vi "writeAPDInfo.vi"(8 "error in (no error)":errorcluster, 9 "iRF Data":cluster{"dt":dbl, "Ctrl V":dbl[], "iRF":dbl[][]}={"dt"=0.0, "Ctrl V"=[0.0], "iRF"=[[0.0]]}, 10 "Gain Data":cluster{"CtrlV":dbl[], "Gain":dbl[]}={"CtrlV"=[0.0], "Gain"=[0.0]}, 11 "APD Serial #":string) -> (0 "error out (no error)":errorcluster)   [LabVIEW 2020]
panel:
  out "appended path":path
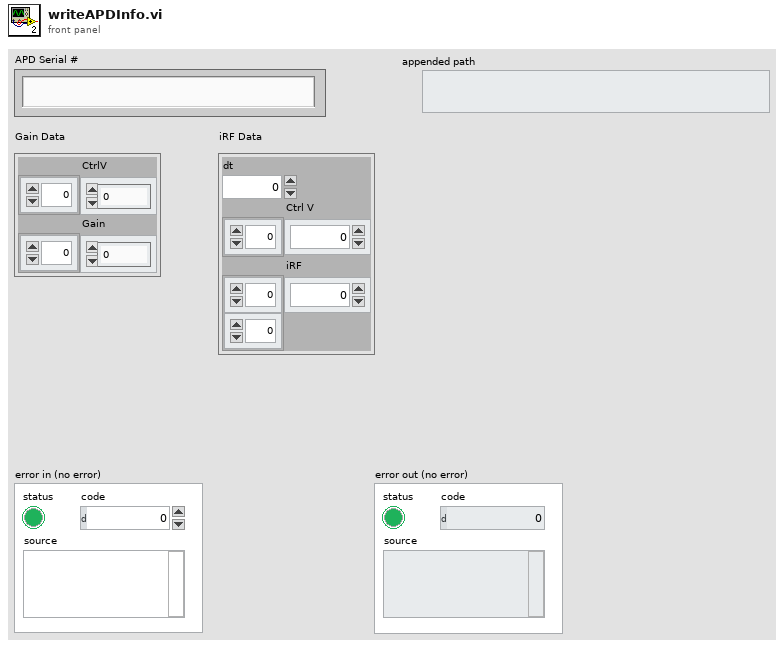
[diagram p1: front panel]
types:
  T1 = enum16{"open", "open or create", "create or replace", "create", "open (read-only)"}
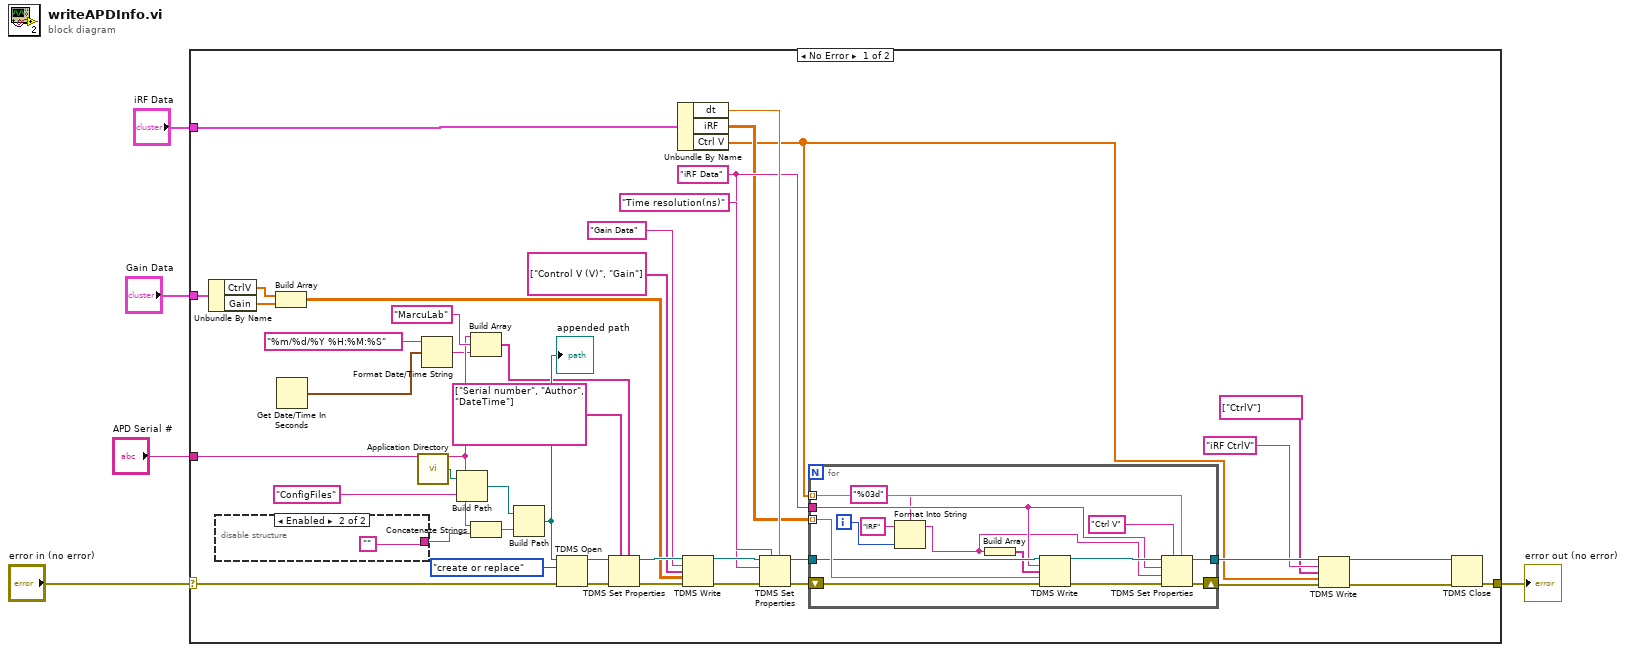
[diagram p0: block diagram]
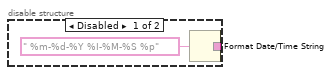
[diagram p2: hidden frame]
diagram:
  n1 = case shown="No Error" "error in (no error)" {
    selector: "error in (no error)" -> [w26 w66]
    tunnel: "APD Serial #" -> [w19 _]
    tunnel: "Gain Data" -> [w35 _]
    tunnel: "iRF Data" -> [w29 _]
    tunnel: [w25 w66] -> w1
    frame No Error {
      w16 = "iRF Data" ("group name in (Untitled)")
      n2 = Unbundle By Name(w35) -> ("CtrlV"=w34:dbl[], "Gain"=w33:dbl[])
      n3 = disable-structure shown="Enabled" {
        disable-tunnel: [w48 ""] -> w20
        frame Disabled {
          n4 = Format Date/Time String(time format string (%c)=" %m-%d-%Y %I-%M-%S %p") -> (date/time string=w48:string)  [unwired: 2 in]
        }
        frame Enabled {
        }
      }
      n5 = Build Array(w34, w33) -> (w32:dbl[][])
      n6 = Get Date/Time In Seconds() -> (seconds since 1Jan1904=w21:timestamp)
      n7 = call <vilib>:"Application Directory.vi"() -> ("Application Directory"=w47:path)
      n8 = Format Date/Time String(time format string (%c)="%m/%d/%Y %H:%M:%S", seconds (now)=w21) -> (date/time string=w17:string)  [unwired: 1 in]
      n9 = Build Path(base path=w47, name or relative path="ConfigFiles") -> (appended path=w45:path)
      n10 = Build Array(w19, "MarcuLab" ("element"), w17) -> (w40:string[])
      n11 = Concatenate Strings(w19, w20) -> (w22:string)
      n12 = Build Path(base path=w45, name or relative path=w22) -> (appended path=w44:path)
      "appended path" <- w44
      n13 = TDMS Open(8:w26, 10:T1."create or replace" ("operation (0:open)"), 11:w44) -> (0:w41:errorcluster, 3:w42:refnum<k34>)  [unwired: 4 in]
      n14 = TDMS Set Properties(5:w40, 7:string[] ["Serial number", "Author", "DateTime"] ("property names"), 8:w41, 11:w42) -> (0:w37:errorcluster, 3:w38:refnum<k34>)  [unwired: 2 in, 2 out]
      n15 = Unbundle By Name(w29) -> ("dt"=w28:dbl, "iRF"=w13:dbl[][], "Ctrl V"=w6:dbl[])
      n16 = TDMS Write(0:w38, 5:"Gain Data" ("group name in (Untitled)"), 7:string[] ["Control V (V)", "Gain"] ("channel name(s) in (Untitled)"), 9:w32, 11:w37) -> (4:w31:refnum<k34>, 15:w30:errorcluster)  [unwired: 1 in, 2 out]
      n17 = TDMS Set Properties(5:w28, 7:"Time resolution(ns)", 8:w30, 10:w16, 11:w31) -> (0:w15:errorcluster, 3:w12:refnum<k34>)  [unwired: 1 in, 2 out]
      n18 = for {
        tunnel: w6 -> [w57] mode=indexing
        tunnel: w16 -> [w58]
        tunnel: [w59] -> w14
        tunnel: w13 -> [w64] mode=indexing
        tunnel: w12 -> [w63]
        shift-right: [w60] -> w10
        shift-left: w15 -> [w65]
        i -> [w51]
        n19 = Format Into String(format string="%03d", initial string="iRF", w51) -> (resulting string=w52:string)  [unwired: 1 in, 1 out]
        n20 = Build Array(w52) -> (w55:string[])
        n21 = TDMS Write(0:w63, 5:w58, 7:w55, 9:w64, 11:w65) -> (4:w62:refnum<k34>, 15:w61:errorcluster)  [unwired: 1 in, 2 out]
        n22 = TDMS Set Properties(5:w57, 7:"Ctrl V", 8:w61, 9:w52, 10:w58, 11:w62) -> (0:w60:errorcluster, 3:w59:refnum<k34>)  [unwired: 2 out]
      }
      n23 = TDMS Write(0:w14, 5:"iRF CtrlV" ("group name in (Untitled)"), 7:string[] ["CtrlV"] ("channel name(s) in (Untitled)"), 9:w6, 11:w10) -> (4:w11:refnum<k34>, 15:w9:errorcluster)  [unwired: 1 in, 2 out]
      n24 = TDMS Close(8:w9, 11:w11) -> (0:w25:errorcluster)  [unwired: 1 out]
    }
    frame Error {
    }
  }
  "error out (no error)" <- w1
